vi "CsTool-CommitAll.vi"(2 "OnlyOnChange (t)":bool=TRUE, 3 "Coerce Flag (f)":bool, 4 "Handle Cluster":T1) -> (0 "Error Code":i32, 1 "Committed":bool)   [LabVIEW 2022 SP3]
doc: "This VI configures a CompuScope system with the configuration settings that are set in the driver. The configuration settings may be set in the driver using the CsTool-ConfigureAcquisition, CsTool-ConfigureChannel, CsTool-ConfigureTrigger, or CsTool-ConfigureTimeStamp VIs. CsTool-Commit.vi must be called in order to actually pass any configuration settings to the CompuScope hardware. The CompuScope system is identified by Handle Cluster, which is obtained with CsTool-GetSystem.vi.\n\nIf set to TRUE, the Coerce flag will coerce all configuration settings to valid available settings for the current CompuScope system. The coercion procedure varies for the different types of configuration settings. For the internal sampling rate, for instance, the coercion procedure chooses the closest available sampling rate. If this flag is set to FALSE, invalid values will not be coerced and the VI will return an error code. The default value is FALSE.\n\nIf set to TRUE, the OnlyOnChange flag will only load configuration settings to the CompuScope hardware if there has been a change to one or more of the settings since the last call to CsTool-Commit.vi. If this flag is set to FALSE, the configuration settings are sent to the CompuScope system even if there have been no changes. The parameter is useful to avoid unnecessary CompuScope system adjustments. The default value is TRUE.\n\nThe Committed output is returned as FALSE if the OnlyOnChange flag is set to TRUE and the settings were unchanged so that no adjustments were performed. Otherwise, it is set to TRUE.\n\nIf the CompuScope hardware was configured correctly by CsTool-Commit.vi, a 1 is returned by the VI. If the return value is 2, the operation was successful but one or more of the settings had to be coerced. Otherwise, an error code is returned. A descriptive error string may be obtained by using CsTool-ErrorHandler.vi."
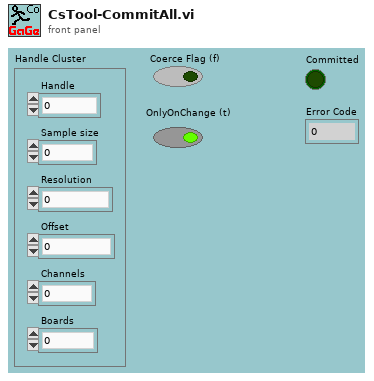
[diagram p1: front panel]
types:
  T1 = cluster{"Handle":u32, "Sample size":u32, "Resolution":i32, "Offset":i32, "Channels":u32, "Boards":u32}
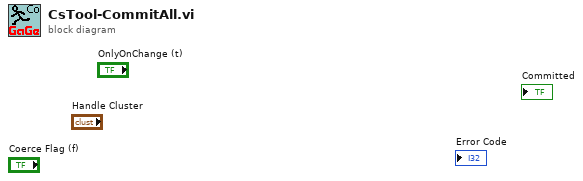
[diagram p0: block diagram]
diagram:
